vi "robot set efg state.vi"(8 "error in (no error)":errorcluster, 9 "distance":sgl, 10 "type":i32, 11 "robot_id":i32) -> (0 "error out":errorcluster)   [LabVIEW 2020]
uses:
  small_scara_interface.dll
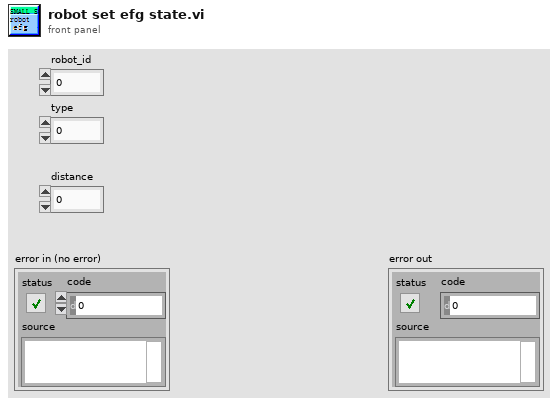
[diagram p1: front panel]
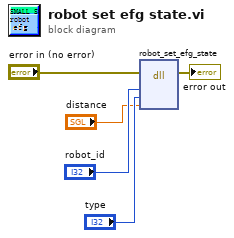
[diagram p0: block diagram]
diagram:
  n1 = dll-call lib="C:/Users/Mogroup-3/Desktop/AutoChem_test/subvi/robot/subvi/Robot-HL/small_scara_interface/small_scara_interface.*" fn="robot_set_efg_state"(error in="error in (no error)", "robot_id"="robot_id", "type"="type", "distance"="distance") -> (error out=→"error out":errorcluster)  [unwired: 6 in, 1 out]
